vi "testPixelFly.vi"() -> ()   [LabVIEW 2009, in "run.lvlib"]
uses:
  testing/run.lvlib
  Tools/Filing/FileNeologist/FileNeologist.lvclass
panel:
  out "Image":T1(plugin-control)
  in  "Save":bool
  out "Board Parameters":T2 {"Vertical bin" items=["1", "2"]; "Horizontal bin" items=["1", "2"]}
  in  "gain":i32(ring) items=["Low (X1)", "High (X2)"]
  in  "exp time":i32(slide)=5 min=1 max=10000 scale=0.0..500.0
  in  "V bin":i32(ring) items=["1", "2"]
  in  "H bin":i32(ring) items=["1", "2"]
  in  "trigger":bool
  in  "Exposure mode":u16(ring)=2 items=["Asynch shutter", "Double shot", "Video mode", "Auto exposure"]
  out "ccdtemp":i32(slide) scale=0.0..100.0
  in  "stop":bool
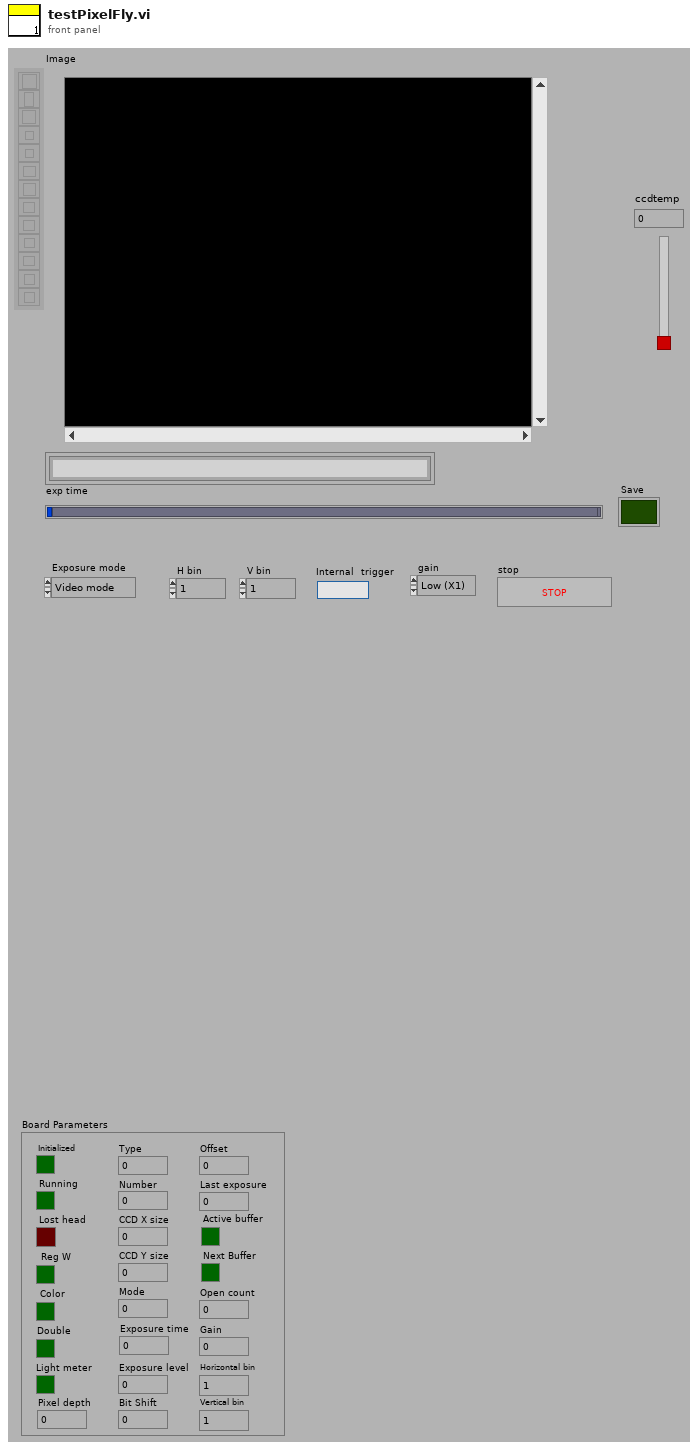
[diagram p1: front panel]
types:
  T1 = typedef "IMAQ Image.ctl" = refnum<image>
  T2 = cluster{"Type":u32, "Number":u32, "Initialized":bool, "Running":bool, "Lost head":bool, "CCD X size":u32, "CCD Y size":u32, "Mode":u32, "Exposure time":u32, "Exposure level":u32, "Horizontal bin":u32, "Vertical bin":u32, "Reg W":bool, "Gain":u32, "Pixel depth":i32, "Bit Shift":u32, "Offset":u32, "Last exposure":u32, "Double ":bool, "Light meter":bool, "Color":bool, "Open count":u32, "Active buffer":bool, "Next Buffer":bool}
  T3 = typedef "IMAQ Rectangle" = cluster{"Left":i32, "Top":i32, "Right":i32, "Bottom":i32, "Rotation":dbl}
  T4 = cluster{"Objects":u16, "Threshold":i32, "Reject Border":bool, "Fill Holes":bool, "Min Object Size":bool, "Min Size":i32, "Max Object Size":bool, "Max Size":i32, "Show Search Area":bool, "Show Center":bool, "Show Bounding Box":bool}
  T5 = cluster{"Left":i32, "Top":i32, "Right":i32, "Bottom":i32}
  T6 = typedef "Image Type" = u32
  T7 = cluster{"ccdxsize":i32, "ccdy":i32, "pictx":i32, "picty":i32, "bitspixel":i32}
  T8 = cluster{"Write":bool, "Write done":bool, "Queued":bool, "Cancelled":bool, "Select":bool, "Select done":bool, "Burst":bool, "Size":bool, "Event":bool, "Timeout":bool, "Open":i32, "Map":i32, "Exposure":i32[], "Offset":i32[], "Size":i32[], "Transfer":i32[], "Total Size":i32}
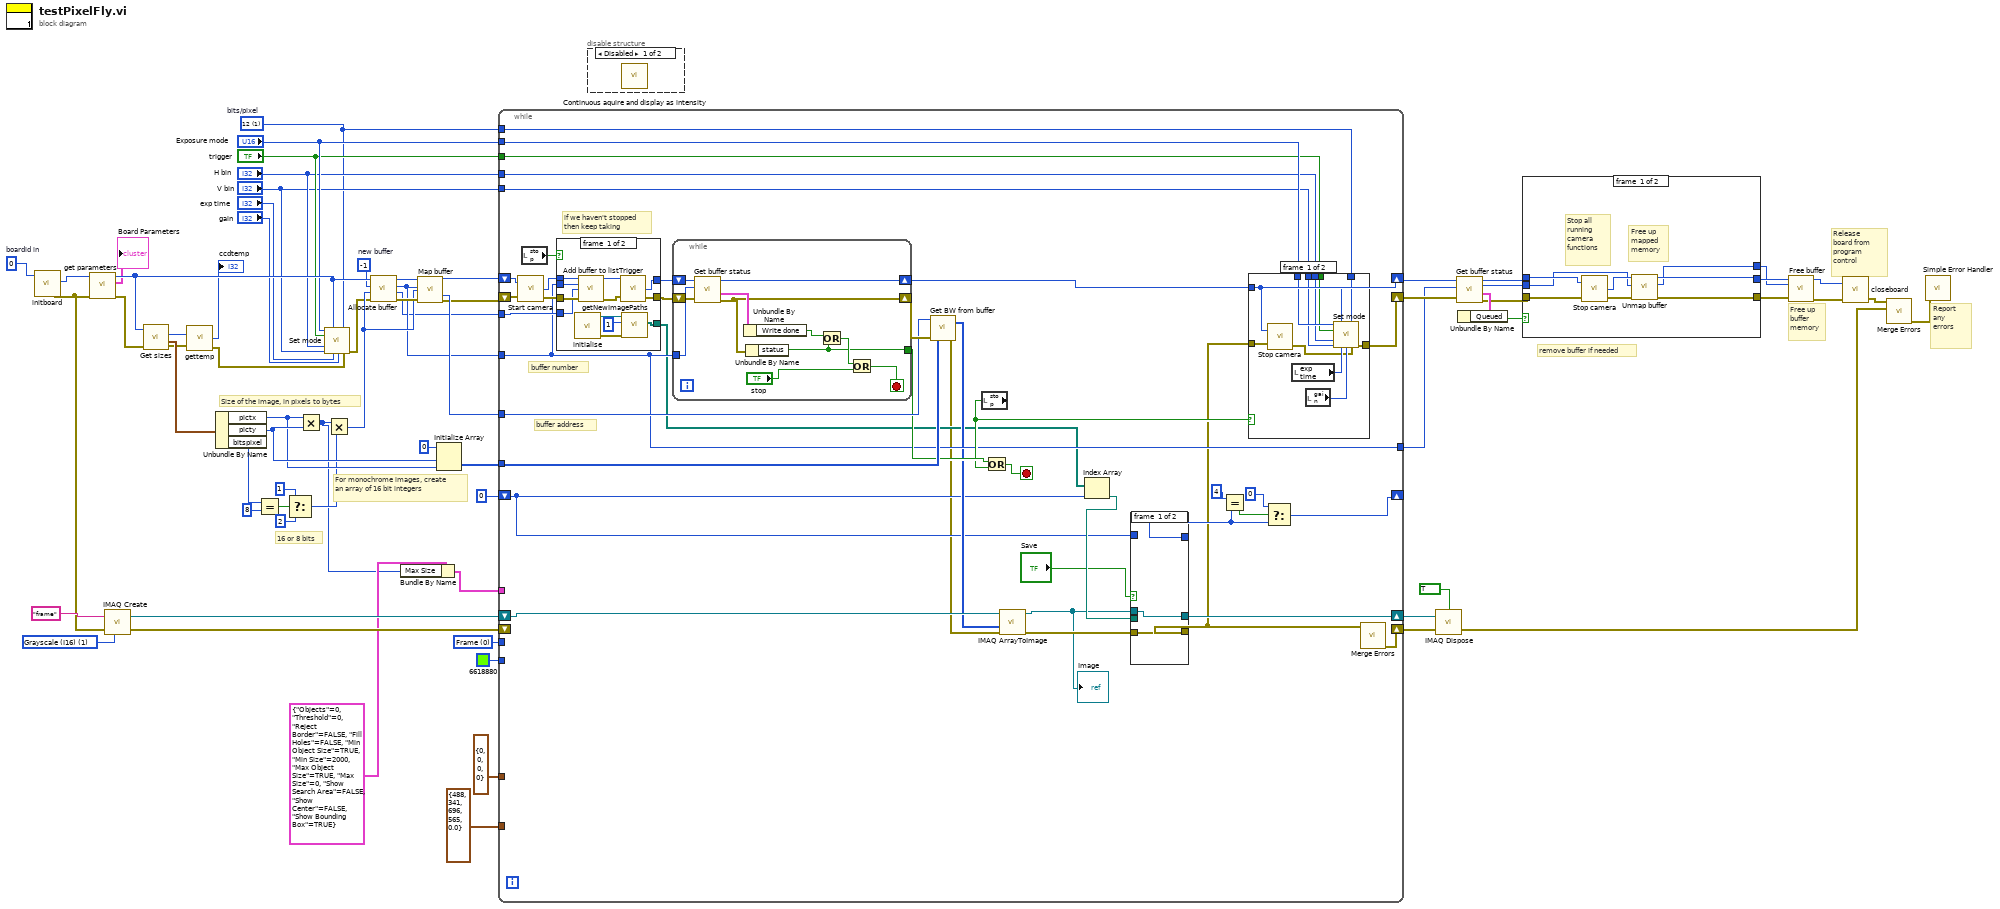
[diagram p0: block diagram]
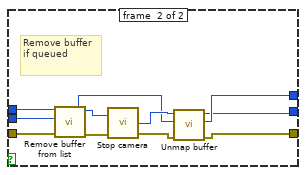
[diagram p3: hidden frame]
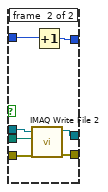
[diagram p4: hidden frame]
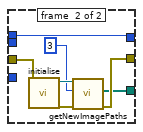
[diagram p6: hidden frame]
diagram:
  w7 = u32 0 items=["Frame", "Fill", "Highlight"] ("Drawing Mode (Frame)")
  w18 = T6 1 items=["Grayscale (U8)", "Grayscale (I16)", "Grayscale (SGL)", "Complex (CSG)", "RGB (U32)", "HSL (U32)", "RGB (U64)", "Grayscale (U16)"] ("Image Type")
  w30 = 1 items=["8", "12"]  # bits/pixel
  w46 = -1  # new buffer
  w51 = 0  # boardid in
  # "remove buffer if needed"
  # "Report any errors"
  # "Release board from program control"
  # "Free up buffer memory"
  # "16 or 8 bits"
  # "For monochrome images, create an array of 16 bit integers"
  # "Size of the image, in pixels to bytes"
  n1 = call <instrlib>:"initboard.vi"("boardid in"=w51) -> ("boardid"=w67:i32, "error out"=w19:errorcluster)  [unwired: 3 in, 1 out]
  n2 = call <instrlib>:"get parameters.vi"("error in (no error)"=w19, "Handle in"=w67) -> ("error out"=w55:errorcluster, "Board Parameters"=→"Board Parameters":T2, "Error out"=w52:i32)  [unwired: 2 in, 1 out]
  n3 = call "IMAQ Create"("Image Name"="frame", "Image Type"=w18, "error in (no error)"=w19) -> ("New Image"=w17:T1, "error out"=w16:errorcluster)  [unwired: 2 in]
  n4 = call <instrlib>:"Get sizes.vi"("Handle in"=w52, "error in (no error)"=w55) -> ("Handle out"=w53:i32, "Picture parameters"=w63:T7, "error out"=w54:errorcluster)  [unwired: 1 in, 1 out]
  n5 = call <instrlib>:"gettemp.vi"("Handle in"=w53, "error in (no error)"=w54) -> ("ccdtemp"=→"ccdtemp":i32, "error out"=w68:errorcluster)  [unwired: 1 out]
  n6 = Unbundle By Name(w63) -> ("pictx"=w60:i32, "picty"=w61:i32, "bitspixel"=w62:i32)
  n7 = Equal?(x=w62, y=8) -> (x = y?=w59:bool)
  n8 = Select(t=1, s=w59, f=2) -> (s? t:f=w56:i32)
  n9 = Multiply(x=w60, y=w61) -> (x*y=w2:i32)
  n10 = call <instrlib>:"Set mode.vi"("Exposure mode"="Exposure mode", "Handle in"=w52, "bits/pixel"=w30, "trigger"="trigger", "H bin"="H bin", "V bin"="V bin", "exp time"="exp time", "gain"="gain", "error in (no error)"=w68) -> ("error out"=w48:errorcluster)  [unwired: 6 in]
  n11 = Multiply(x=w2, y=w56) -> (x*y=w49:i32)
  n12 = call <instrlib>:"Allocate buffer.vi"("error in (no error)"=w48, "Size request"=w49, "Buffer request"=w46, "Handle in"=w52) -> ("error out"=w66:errorcluster, "Size"=w28:i32, "Buffer number"=w29:i32, "Handle out"=w69:i32)
  n13 = Bundle By Name(cluster=T4 {"Objects"=0, "Threshold"=0, "Reject Border"=FALSE, "Fill Holes"=FALSE, "Min Object Size"=TRUE, "Min Size"=2000, "Max Object Size"=TRUE, "Max Size"=0, "Show Search Area"=FALSE, "Show Center"=FALSE, "Show Bounding Box"=TRUE} ("Settings"), "Max Size"=w2) -> (w4:T4)
  n14 = call <instrlib>:"Map buffer.vi"("Handle in"=w69, "Buffer in"=w29, "size"=w49, "error in (no error)"=w66) -> ("Handle out"=w27:i32, "Buffer address"=w50:i32, "error out"=w26:errorcluster)  [unwired: 8 in, 1 out]
  n15 = Initialize Array(u16 0 ("16 bit integers"), w61, w60) -> (w47:u16[][])
  n16 = while {
    tunnel: w29 -> [w88]
    shift-right: [w93] -> w41
    shift-left: w27 -> [w92]
    shift-right: [w94] -> w40
    shift-left: w26 -> [w86]
    tunnel: w50 -> [w104]
    tunnel: w47 -> [w103]
    tunnel: "Exposure mode" -> [w98]
    tunnel: "trigger" -> [w97]
    tunnel: "H bin" -> [w96]
    tunnel: "V bin" -> [w95]
    tunnel: w30 -> [w99]
    tunnel: w28 -> [w102]
    tunnel: [w88] -> w24
    shift-right: [w84] -> w15
    shift-left: w17 -> [w87]
    shift-right: [w85] -> w14
    shift-left: w16 -> [_]
    tunnel: T5 {"Left"=0, "Top"=0, "Right"=0, "Bottom"=0} ("Rectangle") -> [_]
    tunnel: u32 6618880 -> [_]
    tunnel: w7 -> [_]
    tunnel: w4 -> [_]
    tunnel: T3 {"Left"=488, "Top"=341, "Right"=696, "Bottom"=565, "Rotation"=0.0} ("Rectangle") -> [_]
    shift-right: [w79] -> _
    shift-left: 0 -> [w80]
    stop <- w100 stop-if-true
    # "buffer address"
    # "buffer number"
    # "if we haven't stopped\nthen keep taking"
    n17 = call <instrlib>:"Start camera.vi"("Handle in"=w92, "error in (no error)"=w86) -> ("Handle out"=w91:i32, "error out"=w90:errorcluster)  [unwired: 1 out]
    n18 = local read "stop"() -> (w108:bool)
    n19 = case shown="True" w108 {
      tunnel: w90 -> [w141 w144]
      tunnel: [w139 w143] -> w107
      tunnel: w91 -> [w138 w148]
      tunnel: [w136 w148] -> w106
      tunnel: w88 -> [w135 _]
      tunnel: w102 -> [w134 _]
      tunnel: [w131 w142] -> w82
      frame #0 {
        n20 = call "initialise.vi"() -> ("error out"=w132:errorcluster, "FileNeologist out"=w133:refnum<class "FileNeologist.lvclass">)  [unwired: 10 in]
        n21 = call <instrlib>:"Add buffer to list.vi"("Handle in"=w138, "Buffer in"=w135, "size"=w134, "error in (no error)"=w141) -> ("Handle out"=w137:i32, "error out"=w140:errorcluster)  [unwired: 9 in, 1 out]
        n22 = call <instrlib>:"Trigger.vi"("Handle in"=w137, "error in (no error)"=w140) -> ("Handle out"=w136:i32, "error out"=w139:errorcluster)  [unwired: 1 out]
        n23 = call "getNewImagePaths.vi"("error in (no error)"=w132, "numberOfImages"=1, "FileNeologist in"=w133) -> ("Paths"=w131:path[])  [unwired: 6 in, 2 out]
      }
      frame #1 {
        n24 = call "initialise.vi"("error in (no error)"=w144) -> ("error out"=w146:errorcluster, "FileNeologist out"=w147:refnum<class "FileNeologist.lvclass">)  [unwired: 9 in]
        n25 = call "getNewImagePaths.vi"("error in (no error)"=w146, "numberOfImages"=3, "FileNeologist in"=w147) -> ("error out"=w143:errorcluster, "Paths"=w142:path[])  [unwired: 6 in, 1 out]
      }
    }
    n26 = while {
      tunnel: w88 -> [w152]
      shift-right: [w150] -> w93
      shift-left: w106 -> [w153]
      shift-right: [w151] -> w105
      shift-left: w107 -> [w154]
      tunnel: [w149] -> w101
      stop <- w155 stop-if-true
      n27 = call <instrlib>:"Get buffer status.vi"("error in (no error)"=w154, "Buffer request"=w152, "Handle in"=w153) -> ("error out"=w151:errorcluster, "Buffer status"=w159:T8, "Handle out"=w150:i32)  [unwired: 1 in, 1 out]
      n28 = Unbundle By Name(w159) -> ("Write done"=w158:bool)
      n29 = Unbundle By Name(w151) -> ("status"=w149:bool)
      n30 = Or(x=w158, y=w149) -> (x .or. y?=w157:bool)
      n31 = Or(x=w157, y="stop") -> (x .or. y?=w155:bool)
    }
    n32 = call <instrlib>:"Get BW from buffer.vi"("error in (no error)"=w105, "Array input"=w103, "Buffer address"=w104) -> ("error out"=w74:errorcluster, "Image data"=w83:u16[][])
    n33 = local read "stop"() -> (w89:bool)
    n34 = Or(x=w101, y=w89) -> (x .or. y?=w100:bool)
    n35 = call "IMAQ ArrayToImage"("error in (no error)"=w74, "Image Pixels (I16)"=w83, "Image"=w87) -> ("error out"=w73:errorcluster, "Image Out"=w70:T1)  [unwired: 7 in]
    "Image" <- w70
    n36 = Index Array(array=w82, index=w80) -> (element=w81:path)
    n37 = case shown="True" "Save" {
      tunnel: [w110 w117] -> w84
      tunnel: [w109 w116] -> w72
      tunnel: w81 -> [_ w115]
      tunnel: w80 -> [_ w114]
      tunnel: [_ w113] -> w76
      tunnel: w73 -> [w109 w112]
      tunnel: w70 -> [w110 w111]
      frame #0 {
      }
      frame #1 {
        n38 = call-poly "IMAQ Write File 2"("error in (no error)"=w112, "File Path"=w115, "Image"=w111) -> ("error out"=w116:errorcluster, "Image Out (duplicate)"=w117:T1)  [unwired: 7 in]
        n39 = Increment(x=w114) -> (x+1=w113:i32)
      }
    }
    n40 = Equal?(x=4, y=w76) -> (x = y?=w78:bool)
    n41 = case shown="False" w89 {
      tunnel: w99 -> [w128 _]
      tunnel: w98 -> [w127 _]
      tunnel: w97 -> [w126 _]
      tunnel: w96 -> [w125 _]
      tunnel: w95 -> [w124 _]
      tunnel: [w121 w129] -> w94
      tunnel: w72 -> [w120 w129]
      tunnel: w93 -> [w118 _]
      frame #0 {
        n42 = call <instrlib>:"Stop camera.vi"("Handle in"=w118, "error in (no error)"=w120) -> ("error out"=w119:errorcluster)  [unwired: 2 out]
        n43 = local read "exp time"() -> (w123:i32)
        n44 = local read "gain"() -> (w122:i32)
        n45 = call <instrlib>:"Set mode.vi"("Exposure mode"=w127, "Handle in"=w118, "bits/pixel"=w128, "trigger"=w126, "H bin"=w125, "V bin"=w124, "exp time"=w123, "gain"=w122, "error in (no error)"=w119) -> ("error out"=w121:errorcluster)  [unwired: 6 in]
      }
      frame #1 {
      }
    }
    n46 = Select(t=0, s=w78, f=w76) -> (s? t:f=w79:i32)
    n47 = call <vilib>:"Merge Errors.vi"("error in 1 (no error)"=w72) -> ("error out"=w85:errorcluster)  [unwired: 6 in]
  }
  n48 = disable-structure shown="Disabled" {
    frame #0 {
      n49 = call <instrlib>:"Continuous aquire and display as intensity.vi"() -> ()  [unwired: 1 in]
    }
    frame #1 {
    }
  }
  n50 = call "IMAQ Dispose"("All Images? (No)"=TRUE, "Image"=w15, "error in (no error)"=w14) -> ("error out"=w10:errorcluster)  [unwired: 3 in]
  n51 = call <instrlib>:"Get buffer status.vi"("error in (no error)"=w40, "Buffer request"=w24, "Handle in"=w41) -> ("error out"=w42:errorcluster, "Buffer status"=w43:T8, "Buffer number"=w39:i32, "Handle out"=w38:i32)  [unwired: 1 in]
  n52 = Unbundle By Name(w43) -> ("Queued"=w25:bool)
  n53 = case shown="True" w25 {
    tunnel: w42 -> [w164 w178]
    tunnel: [w162 w168] -> w21
    tunnel: w39 -> [w163 w177]
    tunnel: w38 -> [w165 w176]
    tunnel: [w161 w169] -> w23
    tunnel: [w160 w170] -> w22
    frame #0 {
      # "Free up mapped memory"
      # "Stop all running camera functions"
      n54 = call <instrlib>:"Stop camera.vi"("Handle in"=w165, "error in (no error)"=w164) -> ("Handle out"=w167:i32, "error out"=w166:errorcluster)  [unwired: 1 out]
      n55 = call <instrlib>:"Unmap buffer.vi"("error in (no error)"=w166, "Buffer in"=w163, "Handle in"=w167) -> ("error out"=w162:errorcluster, "Buffer number"=w160:i32, "Handle out"=w161:i32)  [unwired: 2 in]
    }
    frame #1 {
      # "Remove buffer if queued"
      n56 = call <instrlib>:"Remove buffer from list.vi"("error in (no error)"=w178, "Buffer in"=w177, "Handle in"=w176) -> ("error out"=w175:errorcluster, "Buffer number"=w171:i32, "Handle out"=w174:i32)  [unwired: 2 in]
      n57 = call <instrlib>:"Stop camera.vi"("Handle in"=w174, "error in (no error)"=w175) -> ("Handle out"=w172:i32, "error out"=w173:errorcluster)  [unwired: 1 out]
      n58 = call <instrlib>:"Unmap buffer.vi"("error in (no error)"=w173, "Buffer in"=w171, "Handle in"=w172) -> ("error out"=w168:errorcluster, "Buffer number"=w170:i32, "Handle out"=w169:i32)  [unwired: 2 in]
    }
  }
  n59 = call <instrlib>:"Free buffer.vi"("error in (no error)"=w21, "Buffer in"=w22, "Handle in"=w23) -> ("error out"=w44:errorcluster, "Handle out"=w37:i32)  [unwired: 2 in, 1 out]
  n60 = call <instrlib>:"closeboard.vi"("Handle in"=w37, "error in (no error)"=w44) -> ("error out"=w12:errorcluster)  [unwired: 2 out]
  n61 = call <vilib>:"Merge Errors.vi"("error in 2 (no error)"=w10, "error in 1 (no error)"=w12) -> ("error out"=w11:errorcluster)  [unwired: 5 in]
  n62 = call <vilib>:"Simple Error Handler.vi"("error in (no error)"=w11) -> ()  [unwired: 4 in, 5 out]
